vi "String.Append Cmd and SubCmd to Message.vi"(7 "Msg":string, 10 "Sub":string, 11 "Cmd":string) -> (3 "Log":string)   [LabVIEW 2018]
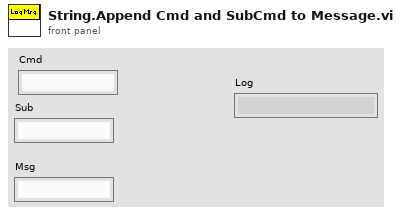
[diagram p1: front panel]
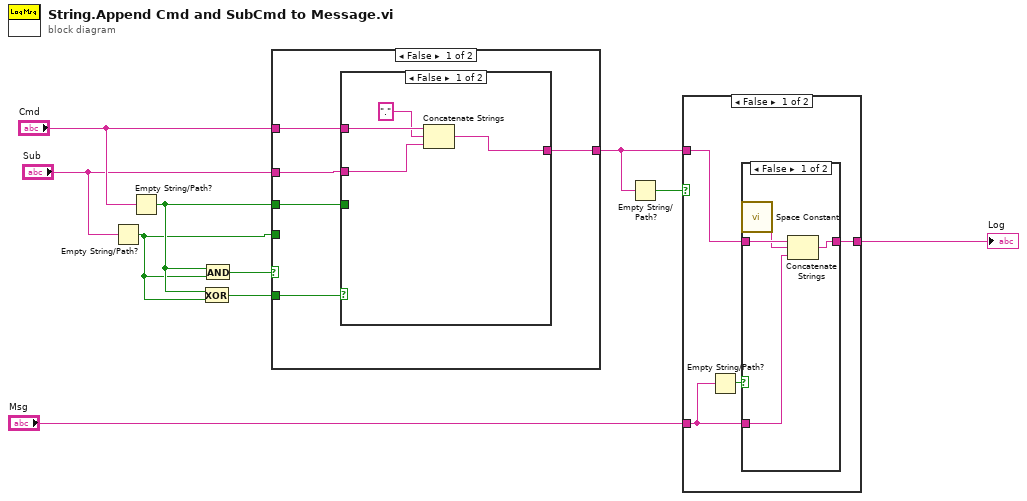
[diagram p0: block diagram]
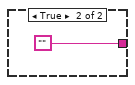
[diagram p6: hidden frame]
diagram:
  n1 = Empty String/Path?(string/path="Sub") -> (empty?=w6:bool)
  n2 = Empty String/Path?(string/path="Cmd") -> (empty?=w7:bool)
  n3 = Exclusive Or(1:w6, 2:w7) -> (0:w5:bool)
  n4 = And(x=w7, y=w6) -> (x .and. y?=w10:bool)
  n5 = case shown="False" w10 {
    tunnel: "Cmd" -> [w14 _]
    tunnel: "Sub" -> [w13 _]
    tunnel: w7 -> [w12 _]
    tunnel: w6 -> [_ _]
    tunnel: [w11 ""] -> w1
    tunnel: w5 -> [w15 _]
    frame False {
      n6 = case shown="False" w15 {
        tunnel: w14 -> [w19 w20]
        tunnel: w13 -> [w17 w21]
        tunnel: w12 -> [_ w23]
        tunnel: [w16 w22] -> w11
        frame False {
          n7 = Concatenate Strings(w19, ".", w17) -> (w16:string)
        }
        frame True {
          n8 = case shown="True" w23 {
            tunnel: [w24 w25] -> w22
            tunnel: w21 -> [_ w25]
            tunnel: w20 -> [w24 _]
            frame False {
            }
            frame True {
            }
          }
        }
      }
    }
    frame True {
    }
  }
  n9 = Empty String/Path?(string/path=w1) -> (empty?=w4:bool)
  n10 = case shown="False" w4 {
    tunnel: [w28 w36] -> w3
    tunnel: "Msg" -> [w27 w36]
    tunnel: w1 -> [w30 _]
    frame False {
      n11 = Empty String/Path?(string/path=w27) -> (empty?=w29:bool)
      n12 = case shown="False" w29 {
        tunnel: w30 -> [w34 w35]
        tunnel: [w33 w35] -> w28
        tunnel: w27 -> [w32 _]
        frame False {
          n13 = call <vilib>:"Space Constant.vi"() -> ("String"=w31:string)
          n14 = Concatenate Strings(w34, w31, w32) -> (w33:string)
        }
        frame True {
        }
      }
    }
    frame True {
    }
  }
  "Log" <- w3
